vi "arraypairmult.vi"() -> ()   [LabVIEW 2022 SP3]
uses:
  <vilib>/numeric/Random Number (Range) U64.vi
  <vilib>/numeric/sub_Random U32.vi
panel:
  out "Array 3":i64[](array[numeric])
  in  "stop":bool
  out "Array 2":i64[](array[numeric])
  out "Array":i64[](array[numeric])
  in  "Numeric":i64
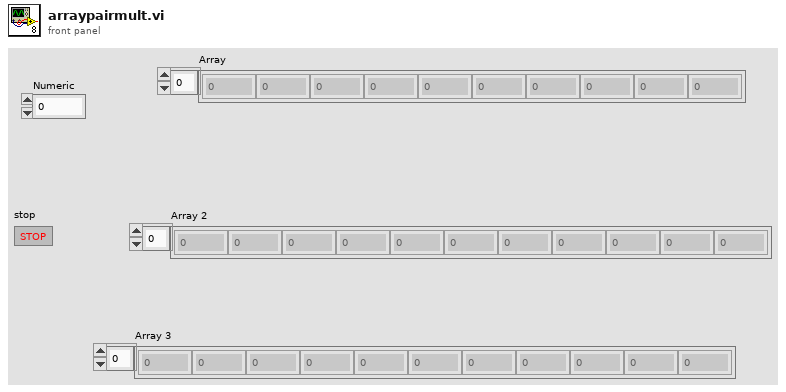
[diagram p1: front panel]
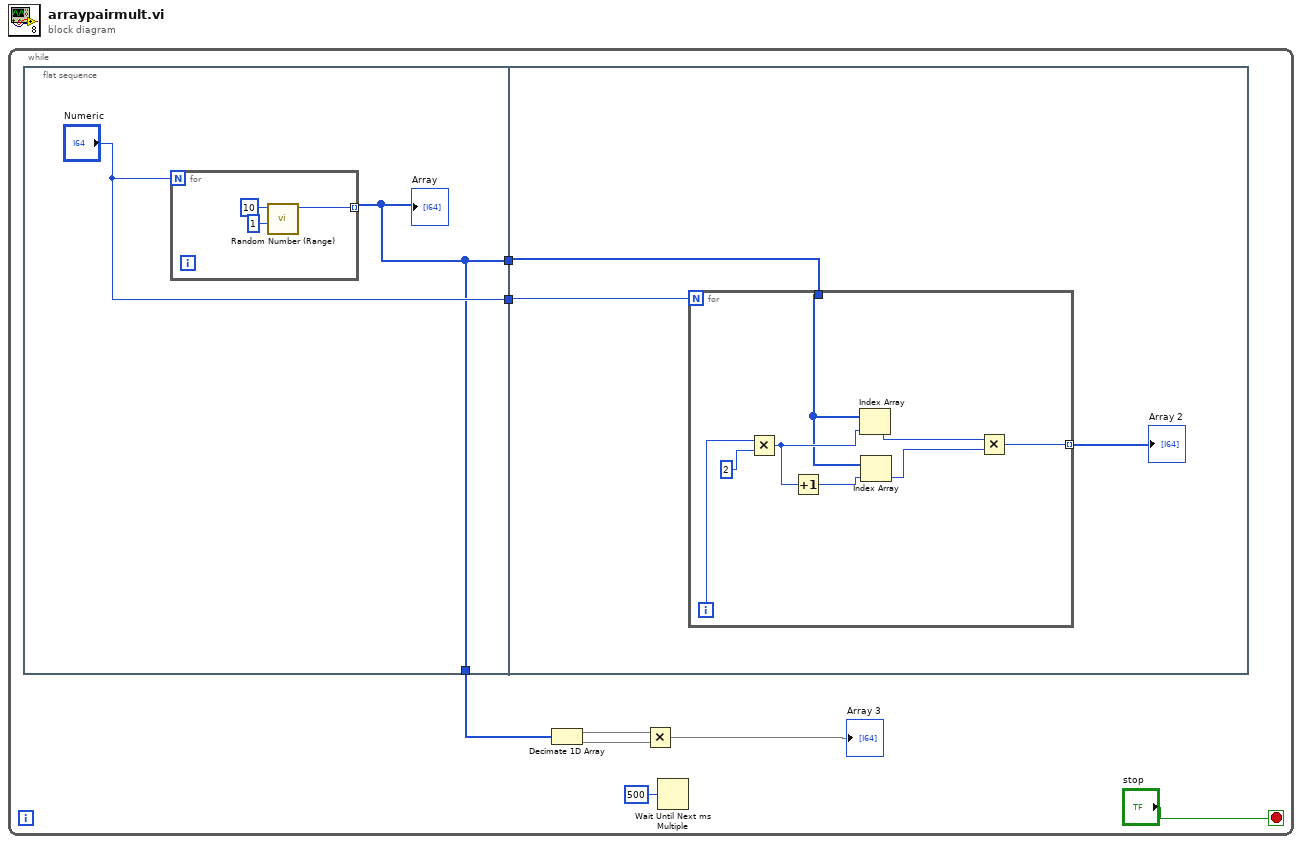
[diagram p0: block diagram]
diagram:
  n1 = while {
    stop <- "stop" stop-if-true
    n2 = flat-sequence {
      tunnel: ["Numeric"] -> w8
      tunnel: [w9] -> w7
      tunnel: [w9] -> w4
      tunnel: w8 -> [w14]
      tunnel: w7 -> [w16]
      frame #0 {
        n3 = for {
          N: "Numeric" -> [_]
          tunnel: [w11] -> w9 mode=indexing
          n4 = call-poly <vilib>:"Random Number (Range).vi"("lower bound (0)"=u64 1, "upper bound (100)"=u64 10) -> ("number"=w11:u64)  [unwired: 9 in]
        }
        "Array" <- w9
      }
      frame #1 {
        n5 = for {
          N: w14 -> [_]
          tunnel: w16 -> [w21]
          tunnel: [w17] -> w15 mode=indexing
          i -> [w18]
          n6 = Multiply(x=w18, y=2) -> (x*y=w23:i32)
          n7 = Increment(x=w23) -> (x+1=w22:i32)
          n8 = Index Array "Index Array"(array=w21, index=w23) -> (element=w20:u64)
          n9 = Index Array(array=w21, index=w22) -> (element=w19:u64)
          n10 = Multiply(x=w20, y=w19) -> (x*y=w17:u64)
        }
        "Array 2" <- w15
      }
    }
    n11 = Decimate 1D Array(w4) -> (w3:u64[], w2:u64[])
    n12 = Multiply(x=w3, y=w2) -> (x*y=→"Array 3":u64[])
    n13 = Wait Until Next ms Multiple(millisecond multiple=u32 500) -> ()  [unwired: 1 out]
  }
